vi "Extract Raw Data.vi"(0 "Host Plot Controls":T1={"refresh"=FALSE, "PMTs for Host"={"Sa"=0, "Sb"=1, "g-factor"=1}, "Peaks"={"# bins"=1000, "min"=0.020751953125, "max"=0.00103759765625}, "Averages"={"# bins"=1000, "max"=0.020751953125, "min"=0.00103759765625}, "Durations"={"# bins"=1000, "max"=20.0, "min"=8.0}, "FP-FPGA"={"# bins"=1000, "max"=20.0, "min"=8.0}, "FP-Host"={"# bins"=1000, "max"=20.0, "min"=8.0}, "Max or Average"=0} {"Max or Average" items=["Peak Max", "Peak Average"]}, 1 "Acquisition rate [Hz]":dbl=100000.0 min=1.0 max=200000.0 step=1.0 format="%#_6p", 2 "subtract baseline?":bool, 7 "FPGA Signal":i32[](array[numeric]), 9 "method":i32(ring)=3 items=["median", "noise center", "Minimum", "lower 20th"], 11 "PMTs to monitor:":T2={"PMT 1"=TRUE, "PMT 2"=TRUE, "PMT 3"=TRUE, "PMT 4"=TRUE}, 12 "display length":i32) -> (3 "Vi(t)":cluster{dbl, dbl, dbl[][]}(graph), 4 "FP(t)":cluster{dbl, dbl, dbl[]}(graph), 6 "Baselines":dbl[](array[numeric]), 8 "raw timetrace data":u32[][](array[numeric]), 10 "raw peaks data":u32[][](array[numeric]), 13 "gains to change":bool[](array[boolean]), 14 "change gains":bool, 15 "Sorting Trace":cluster{dbl, dbl, dbl[]}(graph))   [LabVIEW 2009]
panel:
  out "PMTs for Host":cluster{"Sa":i8, "Sb":i8, "g-factor":i32}
  out "subarray":dbl[](array[numeric])
  out "dt":dbl
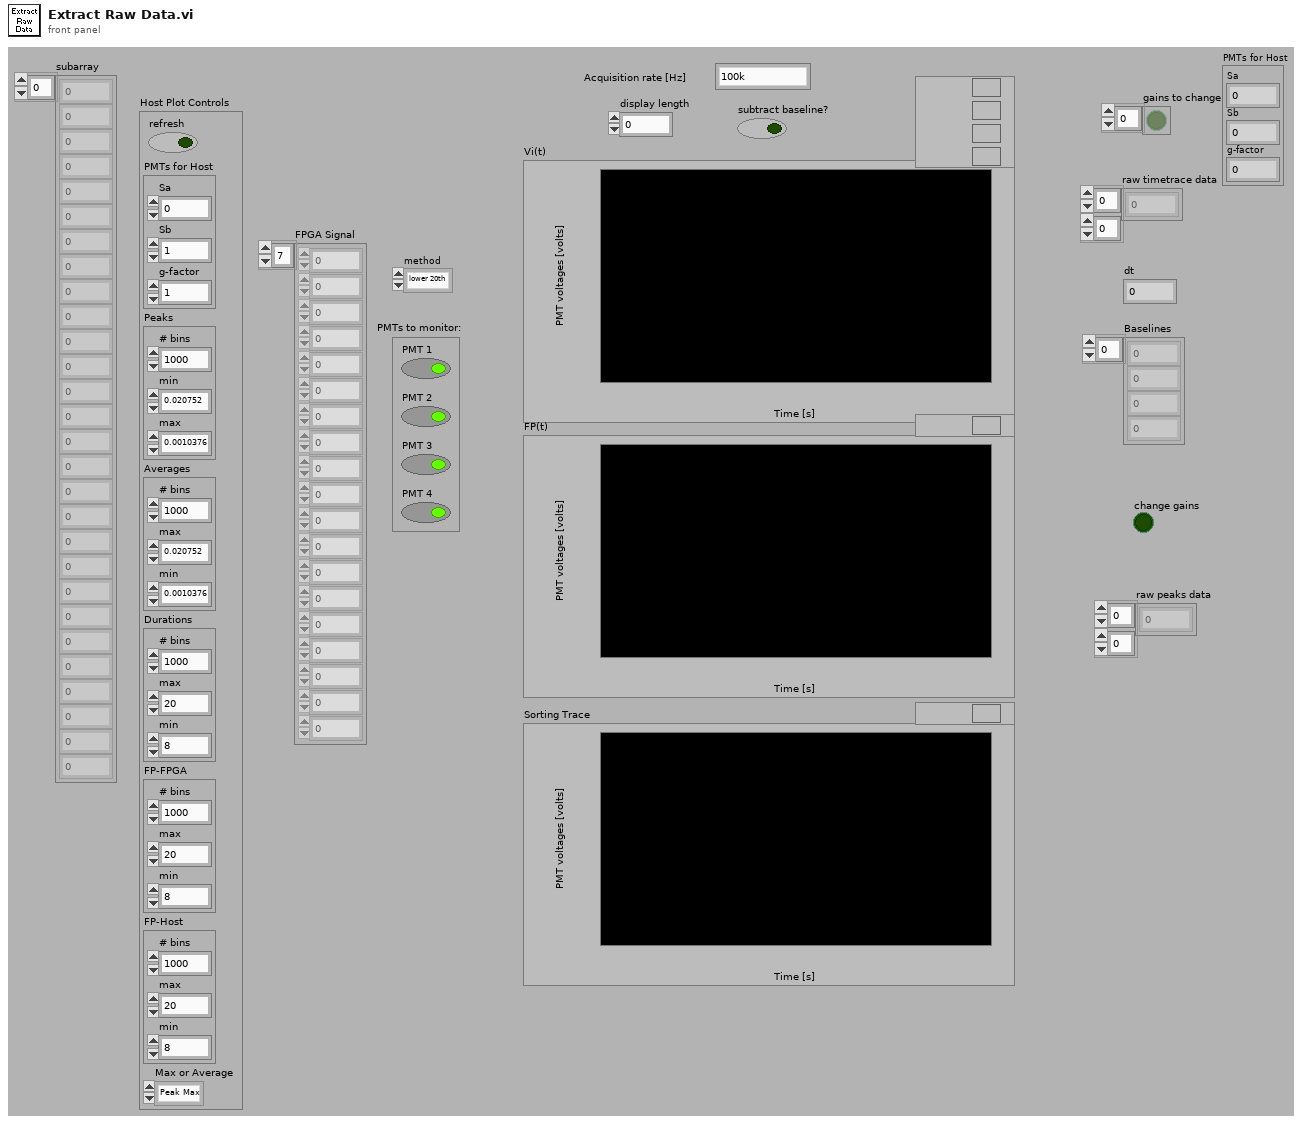
[diagram p1: front panel]
types:
  T1 = cluster{"refresh":bool, "PMTs for Host":cluster{"Sa":i8, "Sb":i8, "g-factor":i32}, "Peaks":cluster{"# bins":i32, "min":dbl, "max":dbl}, "Averages":cluster{"# bins":i32, "max":dbl, "min":dbl}, "Durations":cluster{"# bins":i32, "max":dbl, "min":dbl}, "FP-FPGA":cluster{"# bins":i32, "max":dbl, "min":dbl}, "FP-Host":cluster{"# bins":i32, "max":dbl, "min":dbl}, "Max or Average":i8}
  T2 = cluster{"PMT 1":bool, "PMT 2":bool, "PMT 3":bool, "PMT 4":bool}
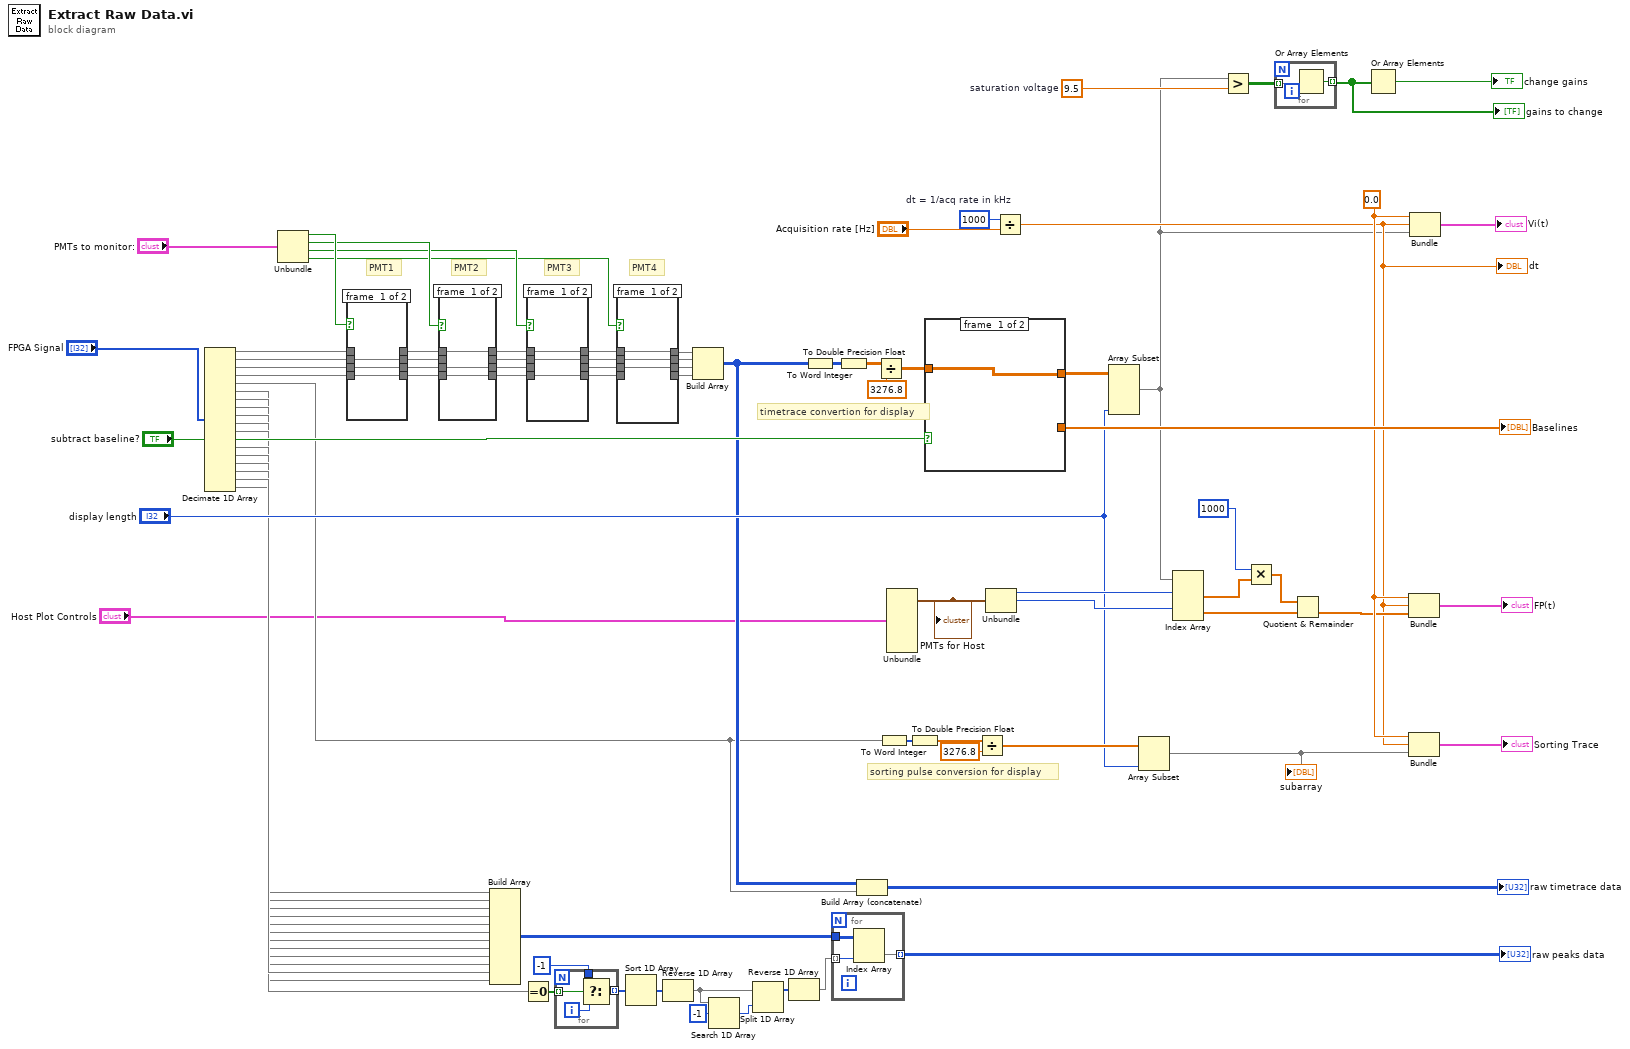
[diagram p0: block diagram]
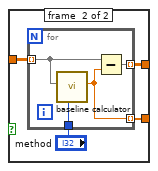
[diagram p6: hidden frame]
diagram:
  w15 = 0.0 ("x/y")
  w83 = 9.5  # saturation voltage
  # "timetrace convertion for display"
  # "sorting pulse conversion for display"
  # "PMT4"
  # "PMT3"
  # "PMT2"
  # "PMT1"
  n1 = Decimate 1D Array("FPGA Signal") -> (w56:i32[], w55:i32[], w54:i32[], w47:i32[], w11:i32[], w30:i32[], w31:i32[], w32:i32[], w33:i32[], w34:i32[], w35:i32[], w36:i32[], w37:i32[], w38:i32[], w39:i32[], w40:i32[], w41:i32[], w9:i32[])
  n2 = Unbundle("PMTs to monitor:") -> ("PMT 1"=w60:bool, "PMT 2"=w59:bool, "PMT 3"=w58:bool, "PMT 4"=w57:bool)
  n3 = case shown="False" w60 {
    tunnel: [_ w94] -> w71
    tunnel: w56 -> [_ w94]
    tunnel: [w90 w93] -> w68
    tunnel: w55 -> [w90 w93]
    tunnel: [w89 w92] -> w65
    tunnel: w54 -> [w89 w92]
    tunnel: w47 -> [w88 w91]
    tunnel: [w88 w91] -> w62
    frame #0 {
    }
    frame #1 {
    }
  }
  n4 = case shown="True" w59 {
    tunnel: [w97 w101] -> w72
    tunnel: w71 -> [w97 w101]
    tunnel: [_ w100] -> w69
    tunnel: w68 -> [_ w100]
    tunnel: [w96 w99] -> w66
    tunnel: w65 -> [w96 w99]
    tunnel: [w95 w98] -> w63
    tunnel: w62 -> [w95 w98]
    frame #0 {
    }
    frame #1 {
    }
  }
  n5 = Build Array(w31, w32, w33, w34, w35, w36, w37, w38, w39, w40, w41, w9) -> (w21:i32[][])
  n6 = Equal To 0?(x=w30) -> (x = 0?=w29:bool[])
  n7 = case shown="True" w58 {
    tunnel: [w102 w108] -> w73
    tunnel: w72 -> [w102 w108]
    tunnel: [w103 w107] -> w70
    tunnel: w69 -> [w103 w107]
    tunnel: [_ w106] -> w67
    tunnel: w66 -> [_ w106]
    tunnel: [w104 w105] -> w64
    tunnel: w63 -> [w104 w105]
    frame #0 {
    }
    frame #1 {
    }
  }
  n8 = for {
    tunnel: w29 -> [w112] mode=indexing
    tunnel: [w111] -> w28 mode=indexing
    tunnel: -1 ("f") -> [w109]
    i -> [w110]
    n9 = Select(t=w109, s=w112, f=w110) -> (s? t:f=w111:i32)
  }
  n10 = case shown="True" w57 {
    tunnel: [w115 w119] -> w53
    tunnel: w73 -> [w115 w119]
    tunnel: [w114 w118] -> w52
    tunnel: w70 -> [w114 w118]
    tunnel: [w113 w117] -> w51
    tunnel: w67 -> [w113 w117]
    tunnel: [_ w116] -> w50
    tunnel: w64 -> [_ w116]
    frame #0 {
    }
    frame #1 {
    }
  }
  n11 = Sort 1D Array(array=w28) -> (sorted array=w27:i32[])
  n12 = Reverse 1D Array(array=w27) -> (reversed array=w24:i32[])
  n13 = Build Array(w53, w52, w51, w50) -> (w12:i32[][])
  n14 = Search 1D Array(1D array=w24, element=-1 ("f")) -> (index of element=w23:i32)  [unwired: 1 in]
  n15 = Split 1D Array(array=w24, index=w23) -> (first subarray=w22:i32[])  [unwired: 1 out]
  n16 = Reverse 1D Array(array=w22) -> (reversed array=w20:i32[])
  n17 = To Word Integer(number=w12) -> (16bit integer=w18:i16[][])
  n18 = for {
    tunnel: w21 -> [w122]
    tunnel: w20 -> [w121] mode=indexing
    tunnel: [w120] -> w19 mode=indexing
    n19 = Index Array(array=w122, index (col)=w121) -> (element=w120:i32[])  [unwired: 1 in]
  }
  "raw peaks data" <- w19
  n20 = To Double Precision Float(number=w18) -> (double precision float=w16:dbl[][])
  n21 = Build Array (concatenate)(w12, w11) -> (→"raw timetrace data":i32[][])
  n22 = Divide(x=w16, y=3276.8) -> (x/y=w46:dbl[][])
  n23 = To Word Integer(number=w11) -> (16bit integer=w14:i16[])
  n24 = Unbundle("Host Plot Controls") -> ("PMTs for Host"=w81:cluster{"Sa":i8, "Sb":i8, "g-factor":i32})  [unwired: 7 out]
  "PMTs for Host" <- w81
  n25 = To Double Precision Float(number=w14) -> (double precision float=w13:dbl[])
  n26 = case shown="True" "subtract baseline?" {
    tunnel: w46 -> [w123 w127]
    tunnel: [w123 w126] -> w42
    tunnel: [_ w125] -> w79
    frame #0 {
    }
    frame #1 {
      n27 = for {
        tunnel: w127 -> [w130] mode=indexing
        tunnel: [w131] -> w126 mode=indexing
        tunnel: [w129] -> w125 mode=indexing
        tunnel: "method" -> [w128]
        n28 = call "baseline calculator.vi"("method"=w128, "timetrace"=w130) -> ("baseline"=w129:dbl)  [unwired: 9 in]
        n29 = Subtract(x=w130, y=w129) -> (x-y=w131:dbl[])
      }
    }
  }
  "Baselines" <- w79
  n30 = Divide(x=w13, y=3276.8) -> (x/y=w45:dbl[])
  n31 = Unbundle(w81) -> ("Sa"=w78:i8, "Sb"=w77:i8)  [unwired: 1 out]
  n32 = Divide "dt = 1/acq rate in kHz"(x=1000, y="Acquisition rate [Hz]") -> (x/y=w3:dbl)
  "dt" <- w3
  n33 = Array Subset(array=w42, length (col)="display length") -> (w2:dbl[][])  [unwired: 3 in]
  n34 = Array Subset(array=w45, length="display length") -> (w44:dbl[])  [unwired: 1 in]
  "subarray" <- w44
  n35 = Index Array(array=w2, index (row) #1=w78, index (row) #2=w77) -> (element #1=w7:dbl[], element #2=w5:dbl[])  [unwired: 2 in]
  n36 = Greater?(x=w2, y=w83) -> (0:w75:bool[][])
  n37 = Multiply(x=1000, y=w7) -> (x*y=w8:dbl[])
  n38 = for {
    tunnel: w75 -> [w133] mode=indexing
    tunnel: [w132] -> w74 mode=indexing
    n39 = Or Array Elements(Boolean array=w133) -> (logical OR=w132:bool)
  }
  "gains to change" <- w74
  n40 = Quotient & Remainder(x=w8, y=w5) -> (floor(x/y)=w4:dbl[])  [unwired: 1 out]
  n41 = Or Array Elements(Boolean array=w74) -> (logical OR=→"change gains":bool)
  n42 = Bundle("x/y"=w15, w3, w4) -> (→"FP(t)":cluster{"x/y":dbl, dbl, dbl[]})  [unwired: 1 in]
  n43 = Bundle("x/y"=w15, w3, w44) -> (→"Sorting Trace":cluster{"x/y":dbl, dbl, dbl[]})  [unwired: 1 in]
  n44 = Bundle("x/y"=w15, w3, w2) -> (→"Vi(t)":cluster{"x/y":dbl, dbl, dbl[][]})  [unwired: 1 in]
